vi "Q8381 Graph scale.vi"(5 "GPIB Address":u16=8, 6 "VISA resource name":refnum<visa-resource-name>) -> (0 "Y max":dbl format="%.5e", 1 "Y min":dbl format="%.5e", 2 "X min":dbl format="%.5e", 3 "X max":dbl format="%.5e", 4 "GPIB Status":bool)   [LabVIEW 2017]
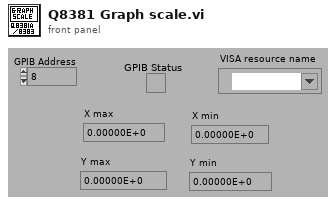
[diagram p1: front panel]
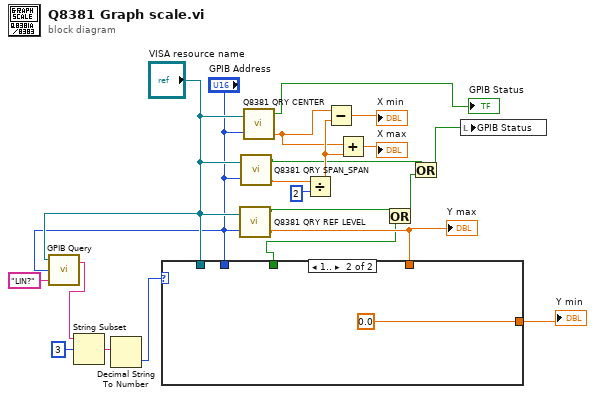
[diagram p0: block diagram]
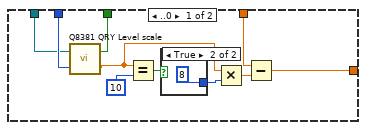
[diagram p2: hidden frame]
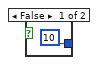
[diagram p3: hidden frame]
diagram:
  n1 = call "GPIB Query.vi"("Command String"="LIN?", "Address"="GPIB Address", "VISA resource name"="VISA resource name") -> ("Query Data"=w1:string)  [unwired: 1 out]
  n2 = String Subset(string=w1, offset (0)=3) -> (substring=w7:string)  [unwired: 1 in]
  n3 = Decimal String To Number(string=w7) -> (number=w6:i32)  [unwired: 2 in, 1 out]
  n4 = call "Q8381 QRY REF LEVEL.vi"("VISA resource name"="VISA resource name", "GPIB Address"="GPIB Address") -> ("GPIB Status"=w10:bool, "REF level value"=w11:ext)  [unwired: 1 out]
  "Y max" <- w11
  n5 = case shown="1.." w6 {
    tunnel: w11 -> [w27 _]
    tunnel: "GPIB Address" -> [w26 _]
    tunnel: [w25 _] -> w9
    tunnel: "VISA resource name" -> [w23 _]
    tunnel: [w22 0.0] -> w5
    frame ..0 {
      n6 = call "Q8381 QRY Level scale.vi"("GPIB address"=w26, "VISA resource name"=w23) -> ("Level value"=w24:sgl, "GPIB status"=w25:bool)
      n7 = Equal?(x=w24, y=10) -> (x = y?=w30:bool)
      n8 = case shown="True" w30 {
        tunnel: [10 8] -> w31
        frame False {
        }
        frame True {
        }
      }
      n9 = Multiply(x=w24, y=w31) -> (x*y=w28:sgl)
      n10 = Subtract(x=w27, y=w28) -> (x-y=w22:ext)
    }
    frame 1.. {
    }
  }
  "Y min" <- w5
  n11 = call "Q8381 QRY SPAN_SPAN.vi"("VISA resource name"="VISA resource name", "GPIB Address"="GPIB Address") -> ("GPIB Status"=w12:bool, "Span value"=w13:dbl)  [unwired: 1 out]
  n12 = call "Q8381 QRY CENTER.vi"("VISA resource name"="VISA resource name", "GPIB Address"="GPIB Address") -> ("GPIB Status"=→"GPIB Status":bool, "Center value"=w14:dbl)  [unwired: 1 out]
  n13 = Divide(x=w13, y=2) -> (x/y=w18:dbl)
  n14 = Subtract(x=w14, y=w18) -> (x-y=→"X min":dbl)
  n15 = Add(x=w14, y=w18) -> (x+y=→"X max":dbl)
  n16 = Or(x=w10, y=w9) -> (x .or. y?=w16:bool)
  n17 = Or(x=w12, y=w16) -> (x .or. y?=w17:bool)
  n18 = local write "GPIB Status"(w17) -> ()
